vi "arrays.vi"() -> ()   [LabVIEW 2024]
panel:
  in  "array":dbl[](array[numeric])
  out "deleted portion":dbl[](array[numeric])
  out "array w/ subset deleted":dbl[](array[numeric])
  out "output array 5":dbl[](array[numeric])
  out "output array 4":dbl[](array[numeric])
  in  "Array to be inserted":dbl[](array[numeric])
  out "output array 3":dbl[](array[numeric])
  out "element 3":dbl
  out "element 2":dbl
  out "element":dbl
  out "size(s)":i32
  out "Array 2":dbl[](array[numeric])
  in  "Array":dbl[](array[numeric])
  out "subarray":dbl[](array[numeric])
  out "min value":dbl
  out "max value":dbl format="%#_13g"
  out "output array 2":dbl[](array[numeric])
  in  "Array 6":dbl[](array[numeric])
  out "output array":dbl[](array[numeric])
  in  "Subarray":dbl[](array[numeric])
  in  "Array 5":dbl[](array[numeric])
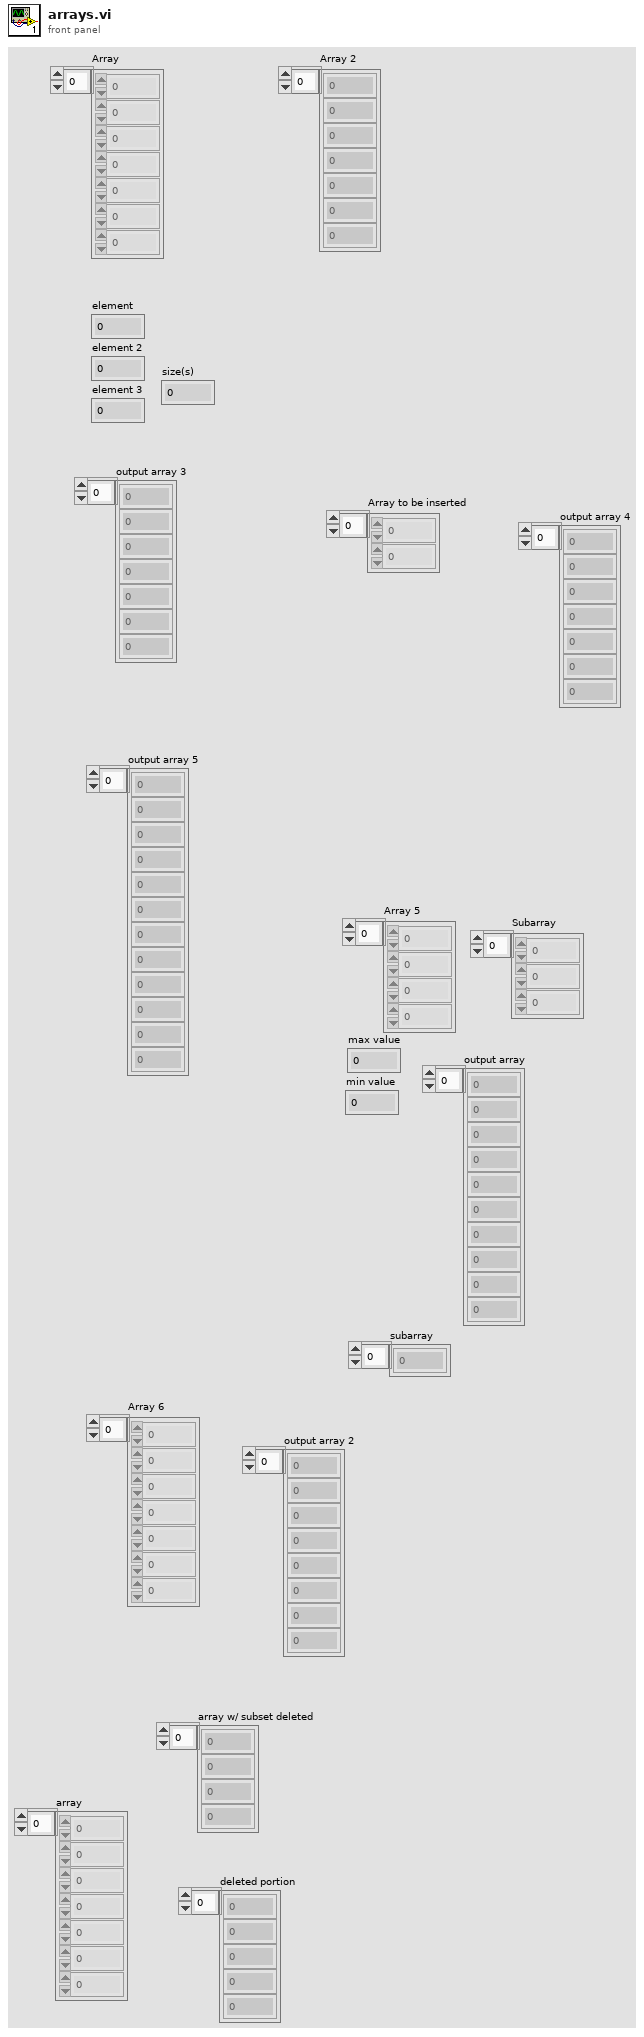
[diagram p1: front panel]
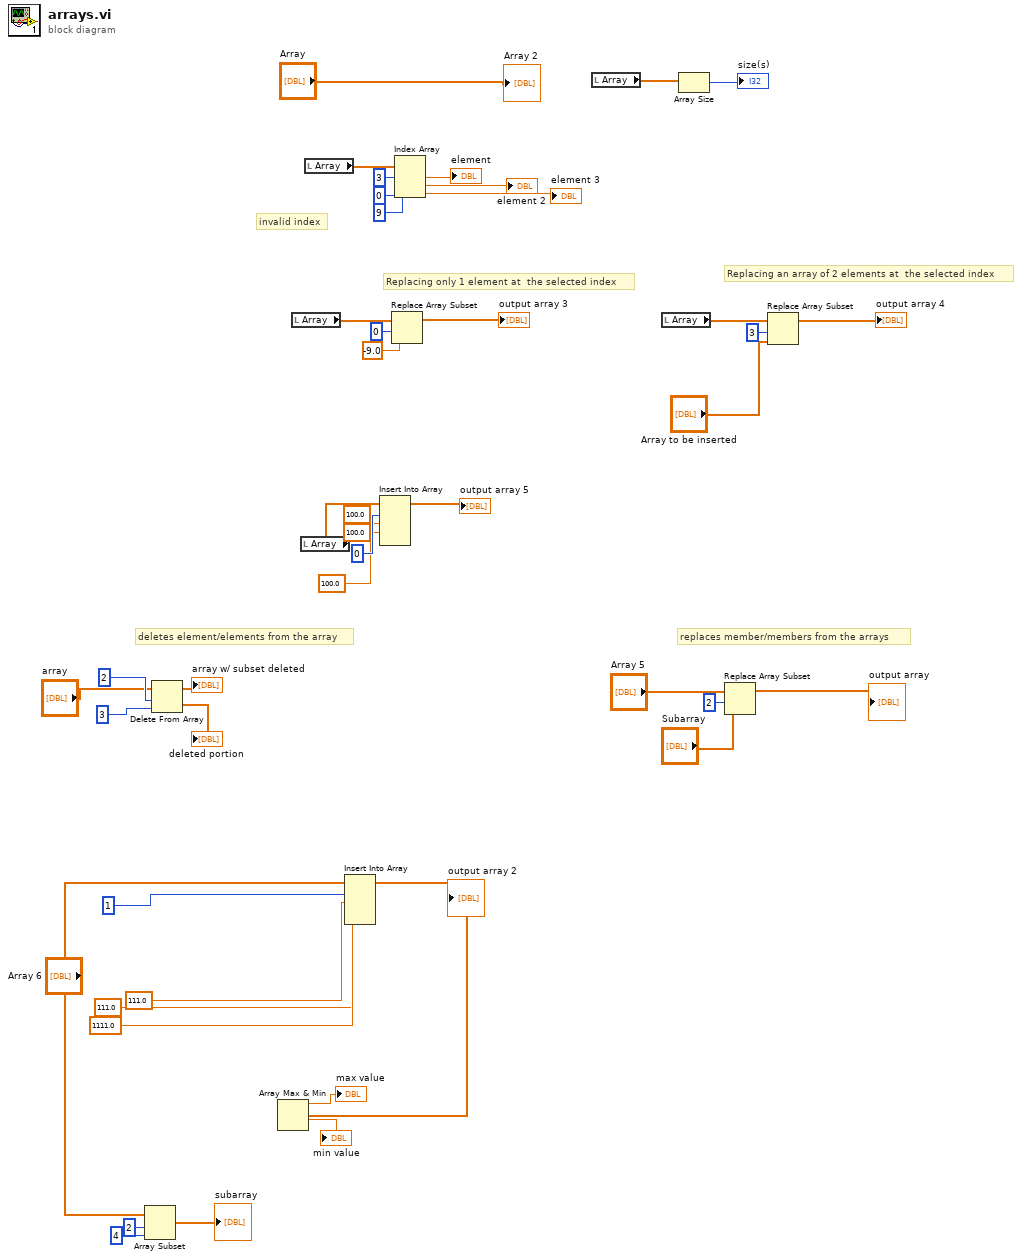
[diagram p0: block diagram]
diagram:
  # "replaces member/members from the arrays"
  # "deletes element/elements from the array"
  # "Replacing an array of 2 elements at  the selected index"
  # "Replacing only 1 element at  the selected index"
  # "invalid index"
  n1 = Array Subset "Array Subset"(array="Array 6", index=2, length=4) -> (→"subarray":dbl[])
  n2 = Delete From Array(array="array", length=2, index=3) -> (deleted portion=→"deleted portion":dbl[], array with subset deleted=→"array w/ subset deleted":dbl[])
  n3 = local read "Array"() -> (w19:dbl[])
  n4 = local read "Array"() -> (w11:dbl[])
  n5 = local read "Array"() -> (w26:dbl[])
  n6 = Insert Into Array "Insert Into Array"(array="Array 6", index=1, new element #1=111.0 ("new element/subarray"), new element #2=111.0 ("new element/subarray"), new element #3=1111.0 ("new element/subarray")) -> (w34:dbl[])
  "output array 2" <- w34
  n7 = Array Max & Min(array=w34) -> (max value=→"max value":dbl, min value=→"min value":dbl)  [unwired: 2 out]
  n8 = Insert Into Array "Insert Into Array"(array=w11, index=0, new element #1=100.0 ("new element/subarray"), new element #2=100.0 ("new element/subarray"), new element #3=100.0 ("new element/subarray")) -> (→"output array 5":dbl[])
  n9 = Replace Array Subset "Replace Array Subset"(array=w19, new element=-9.0 ("new element/subarray"), index=0) -> (→"output array 3":dbl[])
  n10 = Index Array "Index Array"(array=w26, index #1=3 ("index"), index #2=0 ("index"), index #3=9 ("index")) -> (element #1=→"element":dbl, element #2=→"element 2":dbl, element #3=→"element 3":dbl)
  n11 = local read "Array"() -> (w28:dbl[])
  n12 = local read "Array"() -> (w15:dbl[])
  n13 = Array Size(array=w28) -> (size(s)=→"size(s)":i32)
  n14 = Replace Array Subset "Replace Array Subset"(array="Array 5", new element="Subarray", index=2) -> (→"output array":dbl[])
  n15 = Replace Array Subset "Replace Array Subset"(array=w15, new element="Array to be inserted", index=3) -> (→"output array 4":dbl[])
  "Array 2" <- "Array"
